vi "deneyap_tester.vi"() -> ()   [LabVIEW 2016]
panel:
  out "String":string
  out "Start Time":timestamp
  out "Accel Step Count":i32
  out "Gyro Step Count":i32
  out "Test 0":bool
  out "Test 1":bool
  out "Test 2":bool
  out "Test 3":bool
  out "Test 4":bool
  out "Test 5":bool
  out "Test 6":bool
  out "Test 7":bool
  out "Test 8":bool
  out "accel parsed":dbl[](array[numeric])
  out "Accel X":dbl[](graph)
  out "Accel Y":dbl[](graph)
  out "Accel Z":dbl[](graph)
  out "gyro z":dbl[](array[numeric])
  out "gyro y":dbl[](array[numeric])
  out "gyro x":dbl[](array[numeric])
  out "accel z":dbl[](array[numeric])
  out "accel y":dbl[](array[numeric])
  out "accel x":dbl[](array[numeric])
  out "Gyro Z":dbl[](graph)
  out "Gyro Y":dbl[](graph)
  out "Gyro X":dbl[](graph)
  out "gyro parsed":dbl[](array[numeric])
  out "Status":string
  in  "Boolean 2":bool
  in  "Reset":bool
  out "Boolean":bool
  out "Tab Control":T1(tab)
  out "Gpio Memory":bool[](array[boolean])
  out "axis":picture
  out "card_minus_z":picture
  out "card_y":picture
  out "card_x":picture
  out "Accel Steps":enum16{"Wait", "X", "Y", "Z"}(ring)
  out "Gyro Steps":enum16{"Wait", "Constant", "X", "Y", "Z"}(ring)
  out "Gyro Steps":bool[](array[boolean])
  out "Accel Steps":bool[](array[boolean])
  out "Button Memory":bool[](array[boolean])
  out "Instructions":string
  out "Thermometer":dbl(slide) scale=0.0..100.0
  in  "Run Selected Tests":bool
  out "read buffer 2":string
  out "Desired Test":T2(ring)
  in  "stop":bool
  out "Completed Tests":bool[](array[boolean])
  out "Current Operation":enum16{"Timeout", "Read", "Write"}(ring)=enum."Read"
  out "Cluster":T3
  in  "Selected Tests":bool[](array[boolean])
  out "Errors":bool[](array[boolean])
  in  "IMU timeout":dbl=240.0
  in  "IMU Wait":i32=15
  in  "Graph Array Size":i32=30
  in  "GPIO Active Threshold":i32=3000
  in  "Temp. max limit":i32=35
  in  "Temp. min limit":i32=25
  in  "Mic Threshold":i32=3000
  in  "timeout":dbl=60.0
  in  "report save location":path=path "C:/Users/Administrator/Desktop/_deneyap/Deneyap Tester Report.txt"
  in  "VISA resource name 2":refnum<visa-resource-name>="COM4"
  in  "duplicate session (F)":bool
  in  "access mode":u32
  in  "VISA Open timeout (0)":u32
  out "error out":errorcluster
  # "Turn the switch on and run the app, if it is desired to reset the gui"
  # "How to Use ?\n\n- Turn on the reset switch and run the VI, this will reset all values to default.\n- Configure port setting from port settings menu, then choose parameters for the test.\n- Run the VI, then select the tests desired to be performed. After the selection click \"Run Selected Test\" button.\n- Follow the instructions on the instructions box.\n- The green LEDs show which tests are completed and Red LEDs show the tests resulted with errors.\n- In Gyro and Accelometer tests graphs appear on the side of the screen.\n- At the end of the desired tests, a path to save a report will be asked."
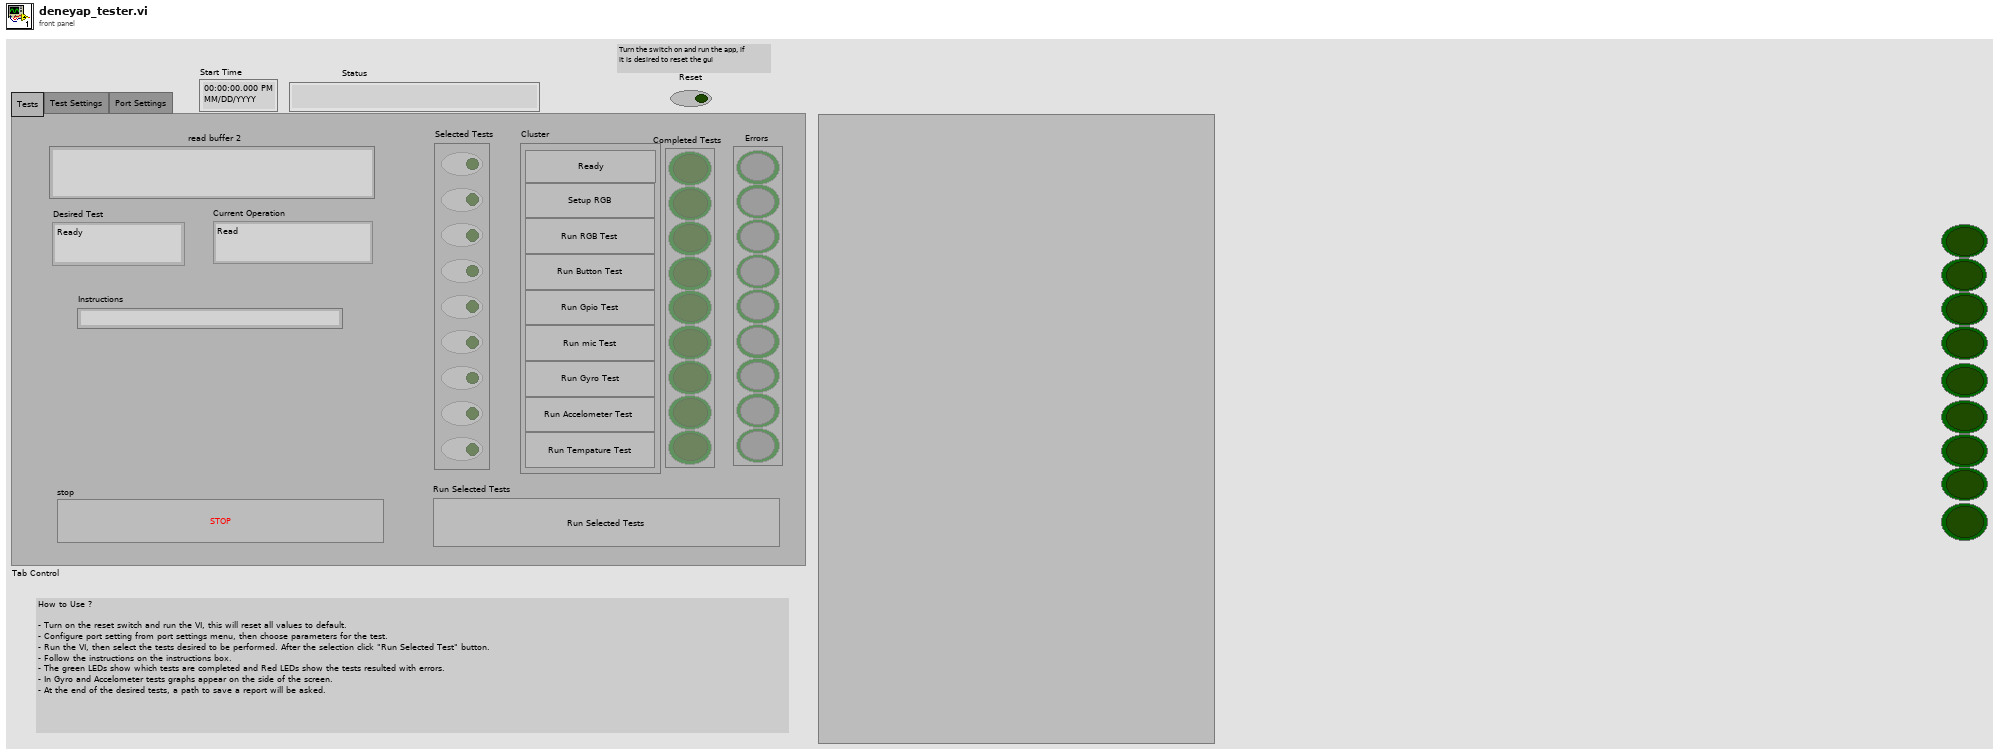
[diagram p1: front panel]
types:
  T1 = enum32{"Tests", "Test Settings", "Port Settings"}
  T2 = enum16{"Ready", "Setup RGB", "Run RGB", "Run button", "Run Gpio", "Run mic", "Run Gyro", "Run Accelometer", "Run Tempature"}
  T3 = cluster{"Ready":bool, "Setup RGB":bool, "Run RGB":bool, "Run Button":bool, "Run Gpio":bool, "Run mic":bool, "Run gyro":bool, "Run Accelometer":bool, "Run tempature":bool}
  T4 = typedef "imagedata.ctl" = cluster{"image type":i32, "image depth":i32, "image":u8[], "mask":u8[], "colors":u32[], "Rectangle":cluster{"left":i16, "top":i16, "right":i16, "bottom":i16}}
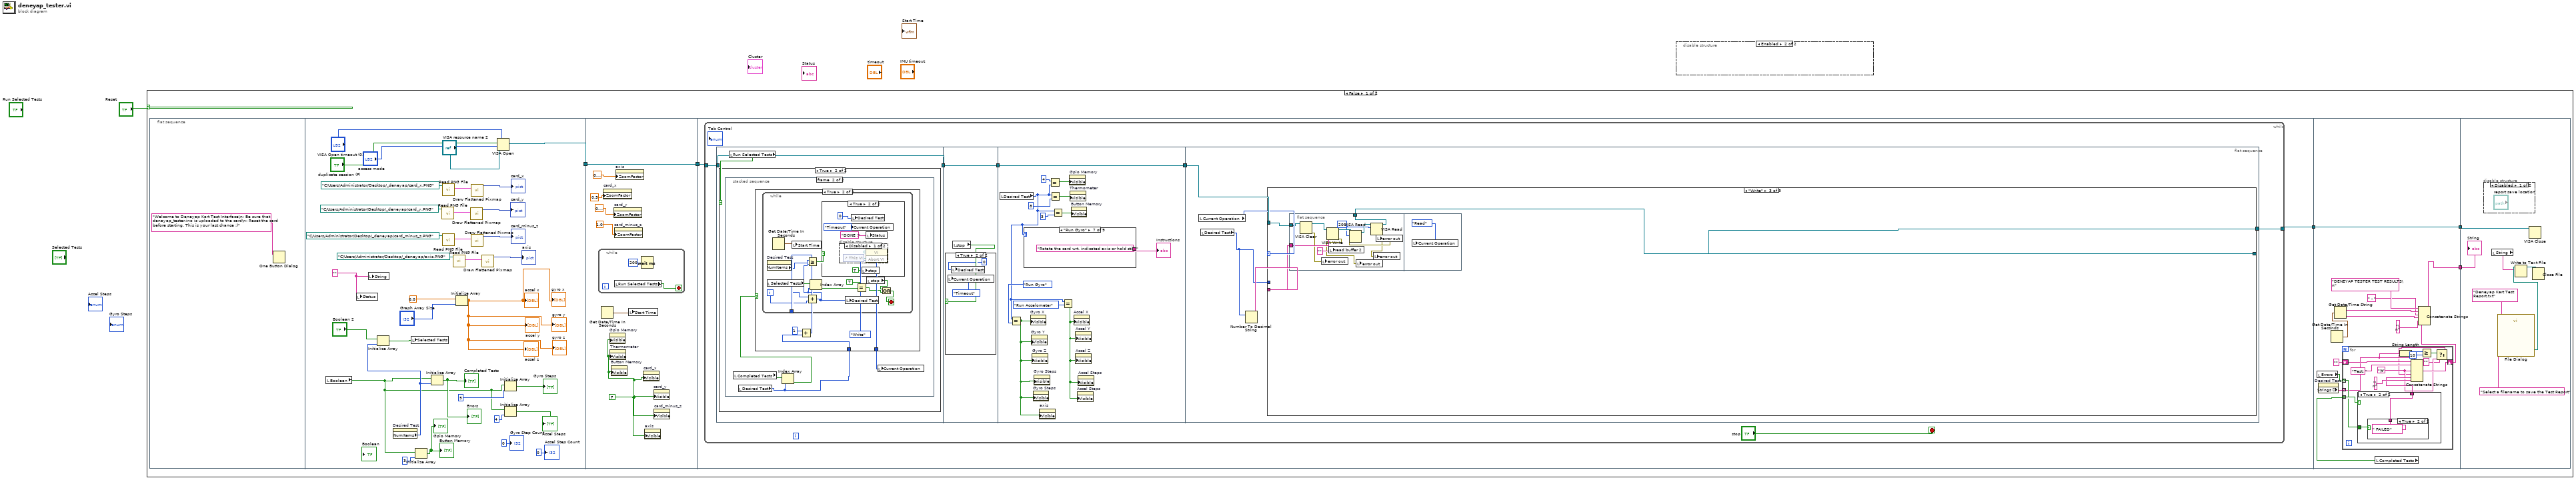
[diagram p0: block diagram]
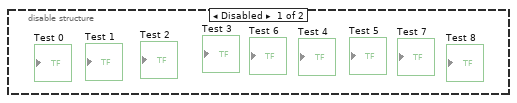
[diagram p2: hidden frame]
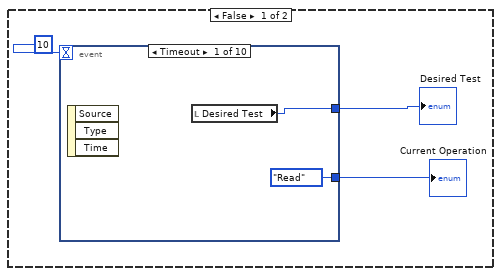
[diagram p3: hidden frame]
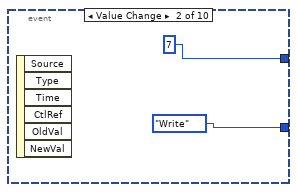
[diagram p4: hidden frame]
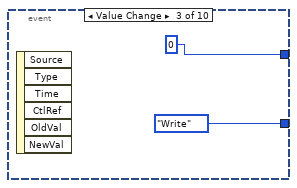
[diagram p5: hidden frame]
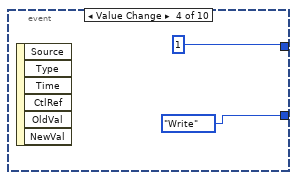
[diagram p6: hidden frame]
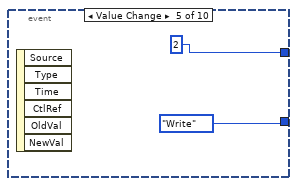
[diagram p7: hidden frame]
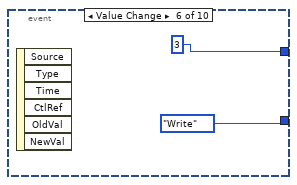
[diagram p8: hidden frame]
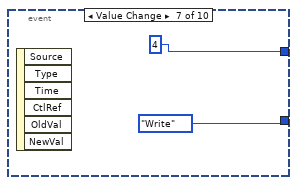
[diagram p9: hidden frame]
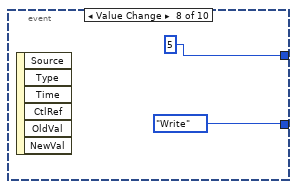
[diagram p10: hidden frame]
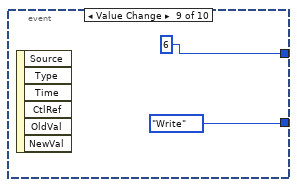
[diagram p11: hidden frame]
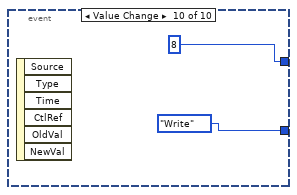
[diagram p12: hidden frame]
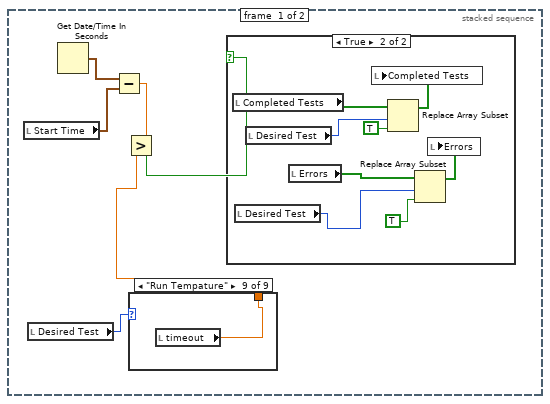
[diagram p13: hidden frame]
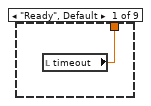
[diagram p14: hidden frame]
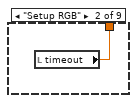
[diagram p15: hidden frame]
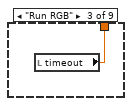
[diagram p16: hidden frame]
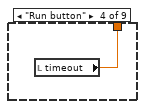
[diagram p17: hidden frame]
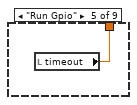
[diagram p18: hidden frame]
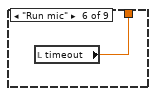
[diagram p19: hidden frame]
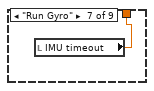
[diagram p20: hidden frame]
diagram:
  n1 = case shown="False" "Reset" {
    frame False {
      n2 = flat-sequence {
        tunnel: [w33] -> w6
        tunnel: w6 -> [w48]
        tunnel: [w48] -> w5
        tunnel: w5 -> [w52]
        tunnel: [w51] -> w4
        tunnel: w4 -> [w526]
        tunnel: [w526] -> w3
        tunnel: [w515] -> w2
        tunnel: w3 -> [w552]
        tunnel: w2 -> [w551]
        frame #0 {
          n3 = One Button Dialog(message="Welcome to Deneyap Kart Test Interface\n- Be sure that denayap_tester.ino is uploaded to the card\n- Reset the card before starting. This is your last chance :)") -> ()  [unwired: 1 in, 1 out]
        }
        frame #1 {
          w8 = ""
          n4 = local read "Boolean"() -> (w24:bool)
          n5 = local write "Status"(w8) -> ()
          n6 = local write "String"(w8) -> ()
          n7 = property on="Desired Test" class="Enum (strict)"() -> ("NumItems"=w36:u32)  [unwired: 2 in, 2 out]
          n8 = Initialize Array("Boolean 2", w36) -> (w35:bool[])
          n9 = local write "Selected Tests"(w35) -> ()
          n10 = Initialize Array(w24, 3) -> (→"Button Memory" →"Gpio Memory":bool[])
          n11 = Initialize Array(w24, w36) -> (→"Completed Tests" →"Errors":bool[])
          n12 = call <vilib>:"Read PNG File.vi"("path to PNG file"=path "C:/Users/Administrator/Desktop/_deneyap/card_y.PNG") -> ("image data"=w17:T4)  [unwired: 8 in, 2 out]
          n13 = call <vilib>:"Read PNG File.vi"("path to PNG file"=path "C:/Users/Administrator/Desktop/_deneyap/card_x.PNG") -> ("image data"=w20:T4)  [unwired: 8 in, 2 out]
          n14 = call <vilib>:"Read PNG File.vi"("path to PNG file"=path "C:/Users/Administrator/Desktop/_deneyap/card_minus_z.PNG") -> ("image data"=w14:T4)  [unwired: 8 in, 2 out]
          n15 = call <vilib>:"Read PNG File.vi"("path to PNG file"=path "C:/Users/Administrator/Desktop/_deneyap/axis.PNG") -> ("image data"=w11:T4)  [unwired: 8 in, 2 out]
          n16 = Initialize Array(0.0 ("element"), "Graph Array Size") -> (→"accel x" →"accel y" →"accel z" →"gyro x" →"gyro y" →"gyro z":dbl[])
          n17 = call <vilib>:"Draw Flattened Pixmap.vi"("image data"=w17) -> ("new picture"=→"card_y":picture)  [unwired: 8 in]
          n18 = call <vilib>:"Draw Flattened Pixmap.vi"("image data"=w20) -> ("new picture"=→"card_x":picture)  [unwired: 8 in]
          n19 = call <vilib>:"Draw Flattened Pixmap.vi"("image data"=w14) -> ("new picture"=→"card_minus_z":picture)  [unwired: 8 in]
          n20 = call <vilib>:"Draw Flattened Pixmap.vi"("image data"=w11) -> ("new picture"=→"axis":picture)  [unwired: 8 in]
          n21 = VISA Open(timeout (0)="VISA Open timeout (0)", duplicate session (F)="duplicate session (F)", access mode="access mode", VISA resource name="VISA resource name 2") -> (VISA resource name=w33:refnum<visa-resource-name>)  [unwired: 1 in, 1 out]
          n22 = Initialize Array(w24, 5 ("dimension size")) -> (→"Gyro Steps":bool[])
          n23 = Initialize Array(w24, 4 ("dimension size")) -> (→"Accel Steps":bool[])
          "Gyro Step Count" <- 0 ("Gyro Step Count")
          "Accel Step Count" <- 0 ("Gyro Step Count")
        }
        frame #2 {
          w42 = FALSE ("Visible")
          n24 = while {
            stop <- w50 stop-if-true
            n25 = local read "Run Selected Tests"() -> (w50:bool)
            n26 = Wait (ms)(milliseconds to wait=u32 200) -> ()  [unwired: 1 out]
          }
          n27 = Get Date/Time In Seconds() -> (seconds since 1Jan1904=w44:timestamp)
          n28 = property on="card_x" class="Pict"("ZoomFactor"=sgl 0.5 ("Zoom Factor")) -> ()  [unwired: 2 in, 2 out]
          n29 = property on="Gpio Memory" class="Arr (strict)"("Visible"=w42) -> ()  [unwired: 2 in, 2 out]
          n30 = property on="Thermometer" class="Slide (strict)"("Visible"=w42) -> ()  [unwired: 2 in, 2 out]
          n31 = property on="Button Memory" class="Arr (strict)"("Visible"=w42) -> ()  [unwired: 2 in, 2 out]
          n32 = property on="card_y" class="Pict"("ZoomFactor"=sgl 0.3 ("Zoom Factor")) -> ()  [unwired: 2 in, 2 out]
          n33 = property on="card_minus_z" class="Pict"("ZoomFactor"=sgl 1.0 ("Zoom Factor")) -> ()  [unwired: 2 in, 2 out]
          n34 = property on="axis" class="Pict"("ZoomFactor"=sgl 0.6 ("Zoom Factor")) -> ()  [unwired: 2 in, 2 out]
          n35 = local write "Start Time"(w44) -> ()
          n36 = property on="card_x" class="Pict"("Visible"=w42) -> ()  [unwired: 2 in, 2 out]
          n37 = property on="axis" class="Pict"("Visible"=w42) -> ()  [unwired: 2 in, 2 out]
          n38 = property on="card_y" class="Pict"("Visible"=w42) -> ()  [unwired: 2 in, 2 out]
          n39 = property on="card_minus_z" class="Pict"("Visible"=w42) -> ()  [unwired: 2 in, 2 out]
        }
        frame #3 {
          n40 = while {
            tunnel: w52 -> [w57]
            tunnel: [w56] -> w51
            stop <- "stop" stop-if-true
            n41 = flat-sequence {
              tunnel: w57 -> [w60]
              tunnel: [w60] -> w54
              tunnel: w54 -> [w134]
              tunnel: [w134] -> w53
              tunnel: w53 -> [w149]
              tunnel: [w149] -> w55
              tunnel: [w162] -> w56
              tunnel: w55 -> [w163]
              frame #0 {
                n42 = local read "Run Selected Tests"() -> (w59:bool)
                n43 = case shown="True" w59 {
                  frame False {
                    n44 = event shown="[0] Timeout" {
                      selector: _ -> [_ _ _ _ _ _ _ _ _ _]
                      dyn-events: _ -> [_ _ _ _ _ _ _ _ _ _]
                      timeout: 10 -> [_ _ _ _ _ _ _ _ _ _]
                      tunnel: [w64 7 0 1 2 3 4 5 6 8] -> w63
                      tunnel: [enum16{"Timeout", "Read", "Write"}."Read" ("Current Operation") enum16{"Timeout", "Read", "Write"}."Write" ("Current Operation") enum16{"Timeout", "Read", "Write"}."Write" ("Current Operation") enum16{"Timeout", "Read", "Write"}."Write" ("Current Operation") enum16{"Timeout", "Read", "Write"}."Write" ("Current Operation") enum16{"Timeout", "Read", "Write"}."Write" ("Current Operation") enum16{"Timeout", "Read", "Write"}."Write" ("Current Operation") enum16{"Timeout", "Read", "Write"}."Write" ("Current Operation") enum16{"Timeout", "Read", "Write"}."Write" ("Current Operation") enum16{"Timeout", "Read", "Write"}."Write" ("Current Operation")] -> w62
                      event Timeout {
                        n45 = event-data() -> ()  [unwired: 1 in, 3 out]
                        n46 = local read "Desired Test"() -> (w64:T2)
                      }
                      event "Cluster.Run Accelometer": Value Change {
                        n47 = event-data() -> ()  [unwired: 1 in, 6 out]
                      }
                      event "Cluster.Ready": Value Change {
                        n48 = event-data() -> ()  [unwired: 1 in, 6 out]
                      }
                      event "Cluster.Setup RGB": Value Change {
                        n49 = event-data() -> ()  [unwired: 1 in, 6 out]
                      }
                      event "Cluster.Run RGB": Value Change {
                        n50 = event-data() -> ()  [unwired: 1 in, 6 out]
                      }
                      event "Cluster.Run Button": Value Change {
                        n51 = event-data() -> ()  [unwired: 1 in, 6 out]
                      }
                      event "Cluster.Run Gpio": Value Change {
                        n52 = event-data() -> ()  [unwired: 1 in, 6 out]
                      }
                      event "Cluster.Run mic": Value Change {
                        n53 = event-data() -> ()  [unwired: 1 in, 6 out]
                      }
                      event "Cluster.Run gyro": Value Change {
                        n54 = event-data() -> ()  [unwired: 1 in, 6 out]
                      }
                      event "Cluster.Run tempature": Value Change {
                        n55 = event-data() -> ()  [unwired: 1 in, 6 out]
                      }
                    }
                    "Current Operation" <- w62
                    "Desired Test" <- w63
                  }
                  frame True {
                    n56 = stacked-sequence {
                      frame #0 {
                        n57 = local read "Start Time"() -> (w88:timestamp)
                        n58 = local read "Desired Test"() -> (w85:T2)
                        n59 = Get Date/Time In Seconds() -> (seconds since 1Jan1904=w89:timestamp)
                        n60 = Subtract(x=w89, y=w88) -> (x-y=w87:dbl)
                        n61 = case shown="\"Run Tempature\"" w85 {
                          tunnel: [w90 w91 w92 w93 w94 w95 w96 w97 w98] -> w84
                          frame "Ready", Default {
                            n62 = local read "timeout"() -> (w90:dbl)
                          }
                          frame "Setup RGB" {
                            n63 = local read "timeout"() -> (w91:dbl)
                          }
                          frame "Run RGB" {
                            n64 = local read "timeout"() -> (w92:dbl)
                          }
                          frame "Run button" {
                            n65 = local read "timeout"() -> (w93:dbl)
                          }
                          frame "Run Gpio" {
                            n66 = local read "timeout"() -> (w94:dbl)
                          }
                          frame "Run mic" {
                            n67 = local read "timeout"() -> (w95:dbl)
                          }
                          frame "Run Gyro" {
                            n68 = local read "IMU timeout"() -> (w96:dbl)
                          }
                          frame "Run Accelometer" {
                            n69 = local read "IMU timeout"() -> (w97:dbl)
                          }
                          frame "Run Tempature" {
                            n70 = local read "timeout"() -> (w98:dbl)
                          }
                        }
                        n71 = Greater?(x=w87, y=w84) -> (0:w86:bool)
                        n72 = case shown="True" w86 {
                          frame False {
                          }
                          frame True {
                            n73 = local read "Completed Tests"() -> (w106:bool[])
                            n74 = local read "Desired Test"() -> (w99:T2)
                            n75 = local read "Desired Test"() -> (w105:T2)
                            n76 = local read "Errors"() -> (w102:bool[])
                            n77 = Replace Array Subset(array=w106, new element=TRUE ("new element/subarray"), index=w105) -> (w103:bool[])
                            n78 = local write "Completed Tests"(w103) -> ()
                            n79 = Replace Array Subset(array=w102, new element=TRUE ("new element/subarray"), index=w99) -> (w101:bool[])
                            n80 = local write "Errors"(w101) -> ()
                          }
                        }
                      }
                      frame #1 {
                        n81 = local read "Completed Tests"() -> (w110:bool[])
                        n82 = local read "Desired Test"() -> (w107:T2)
                        n83 = Index Array(array=w110, index=w107) -> (element=w109:bool)
                        n84 = case shown="True" w109 {
                          tunnel: [enum16{"Timeout", "Read", "Write"}."Read" ("Current Operation") enum16{"Timeout", "Read", "Write"}."Write" ("Current Operation")] -> w108
                          tunnel: w107 -> [_ w114]
                          frame False {
                          }
                          frame True {
                            n85 = Add(x=1, y=w114) -> (x+y=w112:i32)
                            n86 = while {
                              tunnel: w112 -> [w124]
                              i -> [w123]
                              stop <- w118 stop-if-true
                              n87 = property on="Desired Test" class="Enum (strict)"() -> ("NumItems"=w120:u32)  [unwired: 2 in, 2 out]
                              n88 = local read "Selected Tests"() -> (w127:bool[])
                              n89 = Get Date/Time In Seconds() -> (seconds since 1Jan1904=w119:timestamp)
                              n90 = local write "Start Time"(w119) -> ()
                              n91 = Add(x=w124, y=w123) -> (x+y=w121:i32)
                              n92 = Greater Or Equal?(x=w121, y=w120) -> (x >= y?=w122:bool)
                              n93 = Index Array(array=w127, index=w121) -> (element=w126:bool)
                              n94 = case shown="True" w122 {
                                frame False {
                                }
                                frame True {
                                n95 = disable-structure shown="Disabled" {
                                frame Disabled {
                                n96 = control-ref of="This VI"() -> (w132:refnum<vi>)
                                n97 = invoke class="VI" method="Abort VI"(reference=w132) -> ()  [unwired: 2 in, 3 out]
                                }
                                frame Enabled {
                                }
                                }
                                n98 = local write "Current Operation"(enum16{"Timeout", "Read", "Write"}."Timeout" ("Current Operation")) -> ()
                                n99 = local write "Desired Test"(0) -> ()
                                n100 = local write "stop"(TRUE ("stop")) -> ()
                                n101 = local write "Status"("DONE !") -> ()
                                }
                              }
                              n102 = local write "Desired Test"(w121) -> ()
                              n103 = Equal?(x=TRUE, y=w126) -> (x = y?=w117:bool)
                              n104 = local read "stop"() -> (w116:bool)
                              n105 = Or(x=w116, y=w117) -> (x .or. y?=w118:bool)
                            }
                          }
                        }
                        n106 = local write "Current Operation"(w108) -> ()
                      }
                    }
                  }
                }
              }
              frame #1 {
                n107 = local read "stop"() -> (w133:bool)
                n108 = case shown="True" w133 {
                  frame False {
                  }
                  frame True {
                    n109 = local write "Current Operation"(enum16{"Timeout", "Read", "Write"}."Timeout" ("Current Operation")) -> ()
                    n110 = local write "Desired Test"(0) -> ()
                  }
                }
              }
              frame #2 {
                n111 = local read "Desired Test"() -> (w138:T2)
                n112 = Equal?(x=w138, y=T2."Run Gyro") -> (x = y?=w140:bool)
                n113 = case shown="\"Run Gyro\"" w138 {
                  tunnel: ["Ready to start !" "Setting up the RGB" "The RGB LED should blink periodically" "Press on the button" "Make sure that pins are connected properly." "Make some noise to be sure that mic is working" "Rotate the card wrt. indicated axis or hold still " "Hold the card as shown below or hold still" "Checking if the tempature value is between the limits "] -> w146
                  frame "Ready", Default {
                  }
                  frame "Setup RGB" {
                  }
                  frame "Run RGB" {
                  }
                  frame "Run button" {
                  }
                  frame "Run Gpio" {
                  }
                  frame "Run mic" {
                  }
                  frame "Run Gyro" {
                  }
                  frame "Run Accelometer" {
                  }
                  frame "Run Tempature" {
                  }
                }
                "Instructions" <- w146
                n114 = property on="Gyro X" class="WFGraph (strict)"("Visible"=w140) -> ()  [unwired: 2 in, 2 out]
                n115 = property on="Gyro Y" class="WFGraph (strict)"("Visible"=w140) -> ()  [unwired: 2 in, 2 out]
                n116 = property on="Gyro Z" class="WFGraph (strict)"("Visible"=w140) -> ()  [unwired: 2 in, 2 out]
                n117 = property on="Gyro Steps" class="Enum (strict)"("Visible"=w140) -> ()  [unwired: 2 in, 2 out]
                n118 = property on="Gyro Steps" class="Arr (strict)"("Visible"=w140) -> ()  [unwired: 2 in, 2 out]
                n119 = property on="axis" class="Pict"("Visible"=w140) -> ()  [unwired: 2 in, 2 out]
                n120 = Equal?(x=4, y=w138) -> (x = y?=w137:bool)
                n121 = Equal?(x=w138, y=8) -> (x = y?=w147:bool)
                n122 = Equal?(x=w138, y=3) -> (x = y?=w145:bool)
                n123 = Equal?(x=w138, y=T2."Run Accelometer") -> (x = y?=w141:bool)
                n124 = property on="Gpio Memory" class="Arr (strict)"("Visible"=w137) -> ()  [unwired: 2 in, 2 out]
                n125 = property on="Thermometer" class="Slide (strict)"("Visible"=w147) -> ()  [unwired: 2 in, 2 out]
                n126 = property on="Button Memory" class="Arr (strict)"("Visible"=w145) -> ()  [unwired: 2 in, 2 out]
                n127 = property on="Accel X" class="WFGraph (strict)"("Visible"=w141) -> ()  [unwired: 2 in, 2 out]
                n128 = property on="Accel Y" class="WFGraph (strict)"("Visible"=w141) -> ()  [unwired: 2 in, 2 out]
                n129 = property on="Accel Z" class="WFGraph (strict)"("Visible"=w141) -> ()  [unwired: 2 in, 2 out]
                n130 = property on="Accel Steps" class="Enum (strict)"("Visible"=w141) -> ()  [unwired: 2 in, 2 out]
                n131 = property on="Accel Steps" class="Arr (strict)"("Visible"=w141) -> ()  [unwired: 2 in, 2 out]
              }
              frame #3 {
                n132 = local read "Current Operation"() -> (w160:enum16{"Timeout", "Read", "Write"})
                n133 = local read "Desired Test"() -> (w159:T2)
                n134 = Number To Decimal String(number=w159) -> (decimal integer string=w161:string)  [unwired: 1 in]
                n135 = case shown="\"Write\"" w160 {
                  tunnel: w163 -> [w164 w168 w500]
                  tunnel: [w164 w172 w498] -> w162
                  tunnel: w161 -> [_ _ w499]
                  tunnel: w159 -> [_ w167 _]
                  frame "Timeout", Default {
                  }
                  frame "Read" {
                    n136 = VISA Read(VISA resource name=w168, byte count=u32 200) -> (VISA resource name out=w172:refnum<visa-resource-name>, read buffer=→"read buffer 2":string, error out=→"error out":errorcluster)  [unwired: 1 in, 1 out]
                    n137 = disable-structure shown="Enabled" {
                      frame Disabled {
                        n138 = local read "Accel Steps"() -> ()  [unwired: 1 in]
                      }
                      frame Enabled {
                      }
                    }
                    n139 = local read "Completed Tests"() -> (w165:bool[])
                    n140 = case shown="\"Run mic\"" w167 {
                      selector: w167 -> [w176 w179 w185 w211 w233 w250 w265 w390 w488]
                      tunnel: [w174 w178 w183 w210 w232 w251 w263 w381 w487] -> w166
                      tunnel: w165 -> [w175 w180 w184 w209 w230 w249 w264 w389 w485]
                      frame "Ready", Default {
                        n141 = Replace Array Subset(array=w175, new element=TRUE ("new element/subarray"), index=w176) -> (w174:bool[])
                      }
                      frame "Setup RGB" {
                        n142 = Replace Array Subset(array=w180, new element=TRUE ("new element/subarray"), index=w179) -> (w178:bool[])
                      }
                      frame "Run RGB" {
                        n143 = flat-sequence {
                          tunnel: w185 -> [w190]
                          tunnel: w184 -> [w189]
                          tunnel: [w188] -> w182
                          tunnel: w182 -> [w206]
                          tunnel: [w206] -> w181
                          tunnel: [w208] -> w183
                          tunnel: w181 -> [w208]
                          frame #0 {
                            n144 = local read "Errors"() -> (w187:bool[])
                            n145 = Index Array(array=w189, index=w190) -> (element=w191:bool)
                            n146 = case shown="False" w191 {
                              tunnel: w190 -> [w194 _]
                              tunnel: w189 -> [w202 w204]
                              tunnel: [w201 w204] -> w188
                              tunnel: w187 -> [w193 w203]
                              tunnel: [w192 w203] -> w186
                              frame False {
                                n147 = Two Button Dialog(message="Does the RGB LED blink ?\nwith order: white - red - green - blue - cyan - magenta - yellow - no color ", 1:"NO" ("F button name (\"Cancel\")"), 2:"YES" ("T button name (\"OK\")")) -> (T button?=w196:bool)
                                n148 = Replace Array Subset(array=w202, new element=TRUE, index=w194) -> (w201:bool[])
                                n149 = Not(x=w196) -> (.not. x?=w195:bool)
                                n150 = Replace Array Subset(array=w193, new element=w195, index=w194) -> (w192:bool[])
                              }
                              frame True {
                              }
                            }
                            n151 = local write "Errors"(w186) -> ()
                          }
                          frame #1 {
                            n152 = One Button Dialog(message="Reset the card and press the OK button below") -> ()  [unwired: 1 in, 1 out]
                          }
                          frame #2 {
                            n153 = Wait (ms)(milliseconds to wait=u32 200) -> ()  [unwired: 1 out]
                          }
                        }
                      }
                      frame "Run button" {
                        n154 = Index Array(array=w209, index=w211) -> (element=w212:bool)
                        n155 = case shown="False" w212 {
                          tunnel: w209 -> [w227 w229]
                          tunnel: w211 -> [w226 _]
                          tunnel: [w225 w229] -> w210
                          frame False {
                            w214 = 0 ("index")
                            n156 = local read "Button Memory"() -> (w223:bool[])
                            n157 = local read "read buffer 2"() -> (w228:string)
                            n158 = Decimal String To Number(string=w228) -> (number=w224:i32)  [unwired: 2 in, 1 out]
                            n159 = Number To Boolean Array(number=w224) -> (Boolean array=w215:bool[])
                            n160 = Index Array(array=w215, index=w214) -> (element=w213:bool)
                            n161 = Insert Into Array(array=w223, index=w214, new element=w213) -> (w222:bool[])
                            n162 = Delete From Array(array=w222, length=1, index=3) -> (array with subset deleted=w216:bool[])  [unwired: 1 out]
                            n163 = Boolean Array To Number(Boolean array=w216) -> (number=w219:u32)
                            n164 = Equal?(x=w219, y=u32 7) -> (x = y?=w217:bool)
                            n165 = local write "Button Memory"(w216) -> ()
                            n166 = Replace Array Subset(array=w227, new element=w217, index=w226) -> (w225:bool[])
                          }
                          frame True {
                          }
                        }
                      }
                      frame "Run Gpio" {
                        n167 = Index Array(array=w230, index=w233) -> (element=w231:bool)
                        n168 = case shown="False" w231 {
                          tunnel: [w245 w248] -> w232
                          tunnel: w233 -> [w244 _]
                          tunnel: w230 -> [w243 w248]
                          frame False {
                            n169 = local read "read buffer 2"() -> (w246:string)
                            n170 = local read "Gpio Memory"() -> (w239:bool[])
                            n171 = Decimal String To Number(string=w246) -> (number=w242:i32)  [unwired: 2 in, 1 out]
                            n172 = Greater Or Equal?(x=w242, y="GPIO Active Threshold") -> (x >= y?=w240:bool)
                            n173 = Insert Into Array(array=w239, index=0, new element=w240) -> (w238:bool[])
                            n174 = Delete From Array(array=w238, length=1, index=3) -> (array with subset deleted=w234:bool[])  [unwired: 1 out]
                            n175 = And Array Elements(Boolean array=w234) -> (logical AND=w235:bool)
                            n176 = local write "Gpio Memory"(w234) -> ()
                            n177 = Replace Array Subset(array=w243, new element=w235, index=w244) -> (w245:bool[])
                          }
                          frame True {
                          }
                        }
                      }
                      frame "Run mic" {
                        n178 = Index Array(array=w249, index=w250) -> (element=w252:bool)
                        n179 = case shown="False" w252 {
                          tunnel: [w256 w261] -> w251
                          tunnel: w250 -> [w255 _]
                          tunnel: w249 -> [w253 w261]
                          frame False {
                            n180 = local read "read buffer 2"() -> (w257:string)
                            n181 = Decimal String To Number(string=w257) -> (number=w258:i32)  [unwired: 2 in, 1 out]
                            n182 = Absolute Value(x=w258) -> (abs(x)=w259:i32)
                            n183 = Greater Or Equal?(x=w259, y="Mic Threshold") -> (x >= y?=w254:bool)
                            n184 = Replace Array Subset(array=w253, new element=w254, index=w255) -> (w256:bool[])
                          }
                          frame True {
                          }
                        }
                      }
                      frame "Run Gyro" {
                        n185 = flat-sequence {
                          tunnel: [w281] -> w270
                          tunnel: [w280] -> w269
                          tunnel: [w279] -> w268
                          tunnel: [w278] -> w267
                          tunnel: [w277] -> w266
                          tunnel: [w276] -> w262
                          tunnel: w270 -> [w306]
                          tunnel: w269 -> [w305]
                          tunnel: w268 -> [w304]
                          tunnel: w267 -> [w303]
                          tunnel: w266 -> [w302]
                          tunnel: w265 -> [w301]
                          tunnel: w264 -> [w300]
                          tunnel: [w299] -> w263
                          tunnel: w262 -> [w298]
                          frame #0 {
                            n186 = local read "read buffer 2"() -> (w272:string)
                            n187 = Spreadsheet String To Array(delimiter (Tab)=",", format string="%5.3f", spreadsheet string=w272, array type (2D Dbl)=dbl[] []) -> (array=→"gyro parsed":dbl[])
                          }
                          frame #1 {
                            w297 = 0
                            n188 = local read "gyro parsed"() -> (w287:dbl[])
                            n189 = local read "Graph Array Size"() -> (w282:i32)
                            n190 = Index Array(array=w287, index=1) -> (element=w280:dbl)
                            n191 = Index Array(array=w287, index=2) -> (element=w279:dbl)
                            n192 = Index Array(array=w287, index=w297) -> (element=w281:dbl)
                            n193 = local read "gyro z"() -> (w285:dbl[])
                            n194 = local read "gyro y"() -> (w293:dbl[])
                            n195 = local read "gyro x"() -> (w296:dbl[])
                            n196 = Insert Into Array(array=w293, index=0, new element=w280) -> (w291:dbl[])
                            n197 = Insert Into Array(array=w285, index=0, new element=w279) -> (w284:dbl[])
                            n198 = Insert Into Array(array=w296, index=w297, new element=w281) -> (w295:dbl[])
                            n199 = Delete From Array(array=w284, length=1, index=w282) -> (array with subset deleted=w276:dbl[])  [unwired: 1 out]
                            "Gyro Z" <- w276
                            n200 = Delete From Array(array=w291, length=1, index=w282) -> (array with subset deleted=w277:dbl[])  [unwired: 1 out]
                            "Gyro Y" <- w277
                            n201 = Delete From Array(array=w295, length=1, index=w282) -> (array with subset deleted=w278:dbl[])  [unwired: 1 out]
                            "Gyro X" <- w278
                            n202 = local write "gyro y"(w277) -> ()
                            n203 = local write "gyro x"(w278) -> ()
                            n204 = local write "gyro z"(w276) -> ()
                          }
                          frame #2 {
                            n205 = local read "Gyro Steps"() -> (w307:enum16{"Wait", "Constant", "X", "Y", "Z"})
                            n206 = case shown="\"Constant\", Default" w307 {
                              tunnel: w306 -> [_ w327 _ _ _]
                              tunnel: w305 -> [_ w326 _ _ _]
                              tunnel: w304 -> [_ w325 _ _ _]
                              tunnel: w303 -> [_ _ w341 _ _]
                              tunnel: w302 -> [_ _ _ w348 _]
                              tunnel: w301 -> [_ _ _ _ w365]
                              tunnel: w300 -> [w308 w319 w333 w347 w366]
                              tunnel: [w308 w319 w333 w347 w364] -> w299
                              tunnel: w298 -> [_ _ _ _ w361]
                              frame "Wait" {
                                n207 = local read "Gyro Step Count"() -> (w311:i32)
                                n208 = Add(x=w311, y=1) -> (x+y=w312:i32)
                                n209 = local write "Gyro Step Count"(w312) -> ()
                                n210 = Equal?(x=w311, y="IMU Wait") -> (x = y?=w309:bool)
                                n211 = case shown="True" w309 {
                                frame False {
                                }
                                frame True {
                                n212 = local read "Gyro Steps"() -> (w315:bool[])
                                n213 = local write "Gyro Steps"(enum16{"Wait", "Constant", "X", "Y", "Z"}."Constant" ("Gyro Steps")) -> ()
                                n214 = Replace Array Subset(array=w315, new element=TRUE ("new element/subarray"), index=0) -> (w316:bool[])
                                n215 = local write "Gyro Steps"(w316) -> ()
                                }
                                }
                              }
                              frame "Constant", Default {
                                n216 = Equal To 0?(x=w327) -> (x = 0?=w324:bool)
                                n217 = Equal To 0?(x=w326) -> (x = 0?=w323:bool)
                                n218 = Equal To 0?(x=w325) -> (x = 0?=w321:bool)
                                n219 = And(x=w324, y=w323) -> (x .and. y?=w322:bool)
                                n220 = And(x=w322, y=w321) -> (x .and. y?=w320:bool)
                                n221 = case shown="True" w320 {
                                frame False {
                                }
                                frame True {
                                n222 = local read "Gyro Steps"() -> (w329:bool[])
                                n223 = local write "Gyro Steps"(enum16{"Wait", "Constant", "X", "Y", "Z"}."X" ("Gyro Steps")) -> ()
                                n224 = Replace Array Subset(array=w329, new element=TRUE ("new element/subarray"), index=1) -> (w330:bool[])
                                n225 = local write "Gyro Steps"(w330) -> ()
                                }
                                }
                              }
                              frame "X" {
                                n226 = Array Subset(array=w341, index=0, length=5) -> (w338:dbl[])
                                n227 = Absolute Value(x=w338) -> (abs(x)=w337:dbl[])
                                n228 = Greater Or Equal?(x=w337, y=dbl[] [200.0, 200.0, 200.0, 200.0, 200.0]) -> (x >= y?=w335:bool[])
                                n229 = And Array Elements(Boolean array=w335) -> (logical AND=w334:bool)
                                n230 = case shown="True" w334 {
                                frame False {
                                }
                                frame True {
                                n231 = local read "Gyro Steps"() -> (w343:bool[])
                                n232 = local write "Gyro Steps"(enum16{"Wait", "Constant", "X", "Y", "Z"}."Y" ("Gyro Steps")) -> ()
                                n233 = Replace Array Subset(array=w343, new element=TRUE ("new element/subarray"), index=2) -> (w344:bool[])
                                n234 = local write "Gyro Steps"(w344) -> ()
                                }
                                }
                              }
                              frame "Y" {
                                n235 = Array Subset(array=w348, index=0, length=5) -> (w349:dbl[])
                                n236 = Absolute Value(x=w349) -> (abs(x)=w350:dbl[])
                                n237 = Greater Or Equal?(x=w350, y=dbl[] [200.0, 200.0, 200.0, 200.0, 200.0]) -> (x >= y?=w352:bool[])
                                n238 = And Array Elements(Boolean array=w352) -> (logical AND=w351:bool)
                                n239 = case shown="True" w351 {
                                frame False {
                                }
                                frame True {
                                n240 = local read "Gyro Steps"() -> (w357:bool[])
                                n241 = local write "Gyro Steps"(enum16{"Wait", "Constant", "X", "Y", "Z"}."Z" ("Gyro Steps")) -> ()
                                n242 = Replace Array Subset(array=w357, new element=TRUE ("new element/subarray"), index=3) -> (w358:bool[])
                                n243 = local write "Gyro Steps"(w358) -> ()
                                }
                                }
                              }
                              frame "Z" {
                                n244 = Array Subset(array=w361, index=0, length=5) -> (w363:dbl[])
                                n245 = Absolute Value(x=w363) -> (abs(x)=w362:dbl[])
                                n246 = Greater Or Equal?(x=w362, y=dbl[] [200.0, 200.0, 200.0, 200.0, 200.0]) -> (x >= y?=w368:bool[])
                                n247 = And Array Elements(Boolean array=w368) -> (logical AND=w367:bool)
                                n248 = case shown="True" w367 {
                                tunnel: w366 -> [w372 w380]
                                tunnel: w365 -> [_ w379]
                                tunnel: [w372 w377] -> w364
                                frame False {
                                }
                                frame True {
                                n249 = local read "Gyro Steps"() -> (w375:bool[])
                                n250 = Replace Array Subset(array=w380, new element=TRUE, index=w379) -> (w377:bool[])
                                n251 = Replace Array Subset(array=w375, new element=TRUE ("new element/subarray"), index=4) -> (w376:bool[])
                                n252 = local write "Gyro Steps"(w376) -> ()
                                }
                                }
                              }
                            }
                          }
                        }
                      }
                      frame "Run Accelometer" {
                        n253 = flat-sequence {
                          tunnel: [w404] -> w388
                          tunnel: [w403] -> w387
                          tunnel: [w402] -> w386
                          tunnel: [w401] -> w385
                          tunnel: [w400] -> w384
                          tunnel: [w399] -> w383
                          tunnel: [w398] -> w382
                          tunnel: w390 -> [w423]
                          tunnel: w389 -> [w422]
                          tunnel: w388 -> [_]
                          tunnel: w387 -> [_]
                          tunnel: w386 -> [_]
                          tunnel: w385 -> [_]
                          tunnel: w384 -> [_]
                          tunnel: w383 -> [_]
                          tunnel: w382 -> [w421]
                          tunnel: [w420] -> w381
                          frame #0 {
                            n254 = local read "read buffer 2"() -> (w397:string)
                            n255 = Spreadsheet String To Array(delimiter (Tab)=",", format string="%s", spreadsheet string=w397, array type (2D Dbl)=string[] [""]) -> (array=w393:string[])
                            n256 = Fract/Exp String To Number(use system decimal point (T)=FALSE, string=w393) -> (number=→"accel parsed":dbl[])  [unwired: 2 in, 1 out]
                          }
                          frame #1 {
                            w419 = 0
                            n257 = local read "accel parsed"() -> (w398:dbl[])
                            n258 = local read "Graph Array Size"() -> (w405:i32)
                            n259 = Index Array(array=w398, index=1) -> (element=w403:dbl)
                            n260 = Index Array(array=w398, index=2) -> (element=w402:dbl)
                            n261 = Index Array(array=w398, index=w419) -> (element=w404:dbl)
                            n262 = local read "accel z"() -> (w408:dbl[])
                            n263 = local read "accel y"() -> (w415:dbl[])
                            n264 = local read "accel x"() -> (w418:dbl[])
                            n265 = Insert Into Array(array=w415, index=0, new element=w403) -> (w413:dbl[])
                            n266 = Insert Into Array(array=w408, index=0, new element=w402) -> (w407:dbl[])
                            n267 = Insert Into Array(array=w418, index=w419, new element=w404) -> (w417:dbl[])
                            n268 = Delete From Array(array=w407, length=1, index=w405) -> (array with subset deleted=w399:dbl[])  [unwired: 1 out]
                            "Accel Z" <- w399
                            n269 = Delete From Array(array=w413, length=1, index=w405) -> (array with subset deleted=w400:dbl[])  [unwired: 1 out]
                            "Accel Y" <- w400
                            n270 = Delete From Array(array=w417, length=1, index=w405) -> (array with subset deleted=w401:dbl[])  [unwired: 1 out]
                            "Accel X" <- w401
                            n271 = local write "accel y"(w400) -> ()
                            n272 = local write "accel x"(w401) -> ()
                            n273 = local write "accel z"(w399) -> ()
                          }
                          frame #2 {
                            n274 = local read "Accel Steps"() -> (w424:enum16{"Wait", "X", "Y", "Z"})
                            n275 = case shown="\"Z\"" w424 {
                              tunnel: w423 -> [_ _ _ w472]
                              tunnel: w422 -> [w426 w443 w458 w473]
                              tunnel: [w426 w443 w458 w471] -> w420
                              tunnel: w421 -> [_ w441 w456 w469]
                              frame "Wait" {
                                n276 = local read "Accel Step Count"() -> (w428:i32)
                                n277 = local read "IMU Wait"() -> (w425:i32)
                                n278 = Add(x=w428, y=1) -> (x+y=w429:i32)
                                n279 = local write "Accel Step Count"(w429) -> ()
                                n280 = Equal?(x=w428, y=w425) -> (x = y?=w427:bool)
                                n281 = case shown="True" w427 {
                                frame False {
                                }
                                frame True {
                                n282 = local read "Accel Steps"() -> (w433:bool[])
                                n283 = Replace Array Subset(array=w433, new element=TRUE ("new element/subarray"), index=0) -> (w434:bool[])
                                n284 = local write "Accel Steps"(w434) -> ()
                                n285 = local write "Accel Steps"(enum16{"Wait", "X", "Y", "Z"}."X" ("Accel Steps")) -> ()
                                }
                                }
                              }
                              frame "X" {
                                n286 = In Range and Coerce(upper limit=dbl[] [1.1, 0.1, 0.1] ("lower limit"), x=w441, lower limit=dbl[] [0.9, -0.1, -0.1] ("upper limit")) -> (In Range?=w442:bool[])  [unwired: 1 out]
                                n287 = property on="card_x" class="Pict"("Visible"=TRUE) -> ()  [unwired: 2 in, 2 out]
                                n288 = property on="card_y" class="Pict"("Visible"=FALSE) -> ()  [unwired: 2 in, 2 out]
                                n289 = property on="card_minus_z" class="Pict"("Visible"=FALSE) -> ()  [unwired: 2 in, 2 out]
                                n290 = And Array Elements(Boolean array=w442) -> (logical AND=w444:bool)
                                n291 = case shown="False" w444 {
                                frame False {
                                }
                                frame True {
                                n292 = local read "Accel Steps"() -> (w447:bool[])
                                n293 = Replace Array Subset(array=w447, new element=TRUE ("new element/subarray"), index=1) -> (w448:bool[])
                                n294 = local write "Accel Steps"(w448) -> ()
                                n295 = local write "Accel Steps"(enum16{"Wait", "X", "Y", "Z"}."Y" ("Accel Steps")) -> ()
                                }
                                }
                              }
                              frame "Y" {
                                n296 = In Range and Coerce(upper limit=dbl[] [0.1, 1.1, 0.1] ("lower limit"), x=w456, lower limit=dbl[] [-0.1, 0.9, -0.1] ("upper limit")) -> (In Range?=w455:bool[])  [unwired: 1 out]
                                n297 = property on="card_x" class="Pict"("Visible"=FALSE) -> ()  [unwired: 2 in, 2 out]
                                n298 = property on="card_y" class="Pict"("Visible"=TRUE) -> ()  [unwired: 2 in, 2 out]
                                n299 = property on="card_minus_z" class="Pict"("Visible"=FALSE) -> ()  [unwired: 2 in, 2 out]
                                n300 = And Array Elements(Boolean array=w455) -> (logical AND=w457:bool)
                                n301 = case shown="True" w457 {
                                frame False {
                                }
                                frame True {
                                n302 = local read "Accel Steps"() -> (w461:bool[])
                                n303 = local write "Accel Steps"(enum16{"Wait", "X", "Y", "Z"}."Z" ("Accel Steps")) -> ()
                                n304 = Replace Array Subset(array=w461, new element=TRUE ("new element/subarray"), index=2) -> (w462:bool[])
                                n305 = local write "Accel Steps"(w462) -> ()
                                }
                                }
                              }
                              frame "Z" {
                                n306 = In Range and Coerce(upper limit=dbl[] [0.1, 0.1, 1.1] ("lower limit"), x=w469, lower limit=dbl[] [-0.1, -0.1, 0.9] ("upper limit")) -> (In Range?=w470:bool[])  [unwired: 1 out]
                                n307 = And Array Elements(Boolean array=w470) -> (logical AND=w474:bool)
                                n308 = case shown="True" w474 {
                                tunnel: w473 -> [w475 w484]
                                tunnel: w472 -> [_ w483]
                                tunnel: [w475 w481] -> w471
                                frame False {
                                }
                                frame True {
                                n309 = local read "Accel Steps"() -> (w479:bool[])
                                n310 = Replace Array Subset(array=w484, new element=TRUE, index=w483) -> (w481:bool[])
                                n311 = Replace Array Subset(array=w479, new element=TRUE ("new element/subarray"), index=3) -> (w480:bool[])
                                n312 = local write "Accel Steps"(w480) -> ()
                                n313 = property on="card_minus_z" class="Pict"("Visible"=FALSE) -> ()  [unwired: 2 in, 2 out]
                                }
                                }
                                n314 = property on="card_x" class="Pict"("Visible"=FALSE) -> ()  [unwired: 2 in, 2 out]
                                n315 = property on="card_y" class="Pict"("Visible"=FALSE) -> ()  [unwired: 2 in, 2 out]
                                n316 = property on="card_minus_z" class="Pict"("Visible"=TRUE) -> ()  [unwired: 2 in, 2 out]
                              }
                            }
                          }
                        }
                      }
                      frame "Run Tempature" {
                        n317 = Index Array(array=w485, index=w488) -> (element=w486:bool)
                        n318 = case shown="False" w486 {
                          tunnel: [w495 w497] -> w487
                          tunnel: w488 -> [w494 _]
                          tunnel: w485 -> [w493 w497]
                          frame False {
                            n319 = local read "read buffer 2"() -> (w496:string)
                            n320 = Decimal String To Number(string=w496) -> (number=w489:i32)  [unwired: 2 in, 1 out]
                            "Thermometer" <- w489
                            n321 = In Range and Coerce(upper limit="Temp. max limit", x=w489, lower limit="Temp. min limit") -> (In Range?=w490:bool)  [unwired: 1 out]
                            n322 = Replace Array Subset(array=w493, new element=w490, index=w494) -> (w495:bool[])
                          }
                          frame True {
                          }
                        }
                      }
                    }
                    n323 = local write "Completed Tests"(w166) -> ()
                  }
                  frame "Write" {
                    n324 = flat-sequence {
                      tunnel: w500 -> [w511]
                      tunnel: w499 -> [w512]
                      tunnel: [w504] -> w498
                      frame #0 {
                        w503 = u32 200 ("byte count")
                        n325 = VISA Clear(VISA resource name=w511) -> (VISA resource name out=w510:refnum<visa-resource-name>, error out=w506:errorcluster)  [unwired: 1 in]
                        n326 = local write "error out"(w506) -> ()
                        n327 = VISA Write(VISA resource name=w510, write buffer=w512) -> (VISA resource name out=w508:refnum<visa-resource-name>, error out=w501:errorcluster)  [unwired: 1 in, 1 out]
                        n328 = local write "read buffer 2"("" ("read buffer 2")) -> ()
                        n329 = VISA Read(VISA resource name=w508, byte count=w503) -> (VISA resource name out=w505:refnum<visa-resource-name>, error out=w507:errorcluster)  [unwired: 1 in, 2 out]
                        n330 = local write "error out"(w501) -> ()
                        n331 = VISA Read(VISA resource name=w505, byte count=w503) -> (VISA resource name out=w504:refnum<visa-resource-name>, error out=w502:errorcluster)  [unwired: 1 in, 2 out]
                        n332 = local write "error out"(w502) -> ()
                        n333 = local write "error out"(w507) -> ()
                      }
                      frame #1 {
                        n334 = local write "Current Operation"(enum16{"Timeout", "Read", "Write"}."Read" ("Current Operation")) -> ()
                      }
                    }
                  }
                }
              }
            }
          }
        }
        frame #4 {
          n335 = local read "Errors"() -> (w518:bool[])
          n336 = property on="Desired Test" class="Enum (strict)"() -> ("Strings []"=w520:string[])  [unwired: 2 in, 2 out]
          n337 = Get Date/Time In Seconds() -> (seconds since 1Jan1904=w524:timestamp)
          n338 = Get Date/Time String(seconds (now)=w524) -> (date string=w523:string, time string=w521:string)  [unwired: 2 in]
          n339 = local read "Completed Tests"() -> (w519:bool[])
          n340 = for {
            tunnel: w520 -> [w533] mode=indexing
            tunnel: w519 -> [w539] mode=indexing
            tunnel: w518 -> [w536] mode=indexing
            shift-right: [w538] -> w516
            shift-left: "" -> [w537]
            w529 = "\t"
            n341 = case shown="True" w539 {
              tunnel: w536 -> [_ w543]
              tunnel: [" Not Attempted" w542] -> w534
              frame False {
              }
              frame True {
                n342 = case shown="True" w543 {
                  tunnel: [" Completed" " FAILED"] -> w542
                  frame False {
                  }
                  frame True {
                  }
                }
              }
            }
            n343 = String Length(string=w533) -> (length=w532:i32)
            n344 = Greater Or Equal?(x=w532, y=10) -> (x >= y?=w530:bool)
            n345 = Select(t="", s=w530, f=w529) -> (s? t:f=w527:string)
            n346 = Concatenate Strings(w537, "Test: " ("string"), w533, w529, w527, w534, "\n" ("string")) -> (w538:string)
          }
          n347 = Concatenate Strings("DENEYAP TESTER TEST RESULTS\n" ("string"), w523, " - " ("string"), w521, "\n" ("string"), w516) -> (w515:string)
        }
        frame #5 {
          n348 = disable-structure shown="Disabled" {
            frame Disabled {
            }
            frame Enabled {
            }
          }
          n349 = local read "String"() -> (w546:string)
          n350 = call "File Dialog"("prompt"="Select a filename to save the Test Report", "default name"="Deneyap Kart Test Report.txt") -> ("selected path"=w547:path)  [unwired: 10 in, 3 out]
          n351 = Write to Text File(file (use dialog)=w547, text=w546) -> (refnum out=w550:refnum<file>)  [unwired: 2 in, 2 out]
          n352 = VISA Close(VISA resource name=w552) -> ()  [unwired: 1 in, 1 out]
          n353 = Close File(refnum=w550) -> ()  [unwired: 1 in, 2 out]
          "String" <- w551
        }
      }
    }
    frame True {
      n354 = control-ref of="This VI"() -> (w553:refnum<vi>)
      n355 = invoke class="VI" method="Default Vals.Reinit All"(reference=w553) -> ()  [unwired: 2 in, 3 out]
    }
  }
  n356 = disable-structure shown="Enabled" {
    frame Disabled {
    }
    frame Enabled {
    }
  }
